vi "Test_Aerotech.vi"() -> ()   [LabVIEW 2009]
uses:
  Controls/AerotechTarget.ctl
panel:
  in  "Velocity":dbl
  in  "Position":dbl
  out "AEROTECH.ACTUAL":T1
  in  "stop":bool
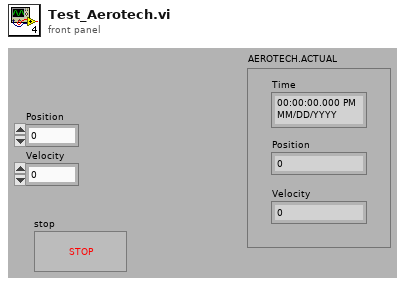
[diagram p1: front panel]
types:
  T1 = typedef "AerotechTarget.ctl" = cluster{"Time":timestamp, "Position":dbl, "Velocity":dbl}
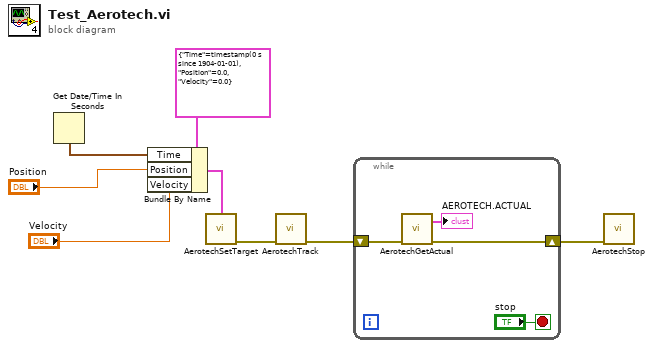
[diagram p0: block diagram]
diagram:
  n1 = Get Date/Time In Seconds() -> (seconds since 1Jan1904=w3:timestamp)
  n2 = Bundle By Name(cluster=T1 {"Time"=timestamp(0 s since 1904-01-01), "Position"=0.0, "Velocity"=0.0} ("AEROTECH.TARGET"), "Time"=w3, "Position"="Position", "Velocity"="Velocity") -> (w5:T1)
  n3 = call "AerotechSetTarget.vi"("AEROTECH.TARGET"=w5) -> ("error out"=w8:errorcluster)  [unwired: 4 in]
  n4 = call "AerotechTrack.vi"("error in (no error)"=w8) -> ("error out"=w7:errorcluster)  [unwired: 10 in]
  n5 = while {
    shift-right: [w10] -> w6
    shift-left: w7 -> [w12]
    stop <- "stop" stop-if-true
    n6 = call "AerotechGetActual.vi"("error in (no error)"=w12) -> ("error out"=w10:errorcluster, "AEROTECH.ACTUAL"=→"AEROTECH.ACTUAL":T1)  [unwired: 3 in]
  }
  n7 = call "AerotechStop.vi"("error in (no error)"=w6) -> ()  [unwired: 10 in, 1 out]
